vi "ADDER.vi"(2 "INPUT2":bool, 3 "INPUT1":bool) -> (0 "CARRY":bool, 1 "SUM":bool)   [LabVIEW 2017]
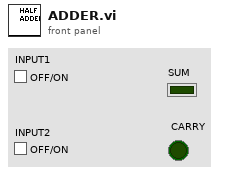
[diagram p1: front panel]
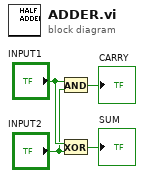
[diagram p0: block diagram]
diagram:
  n1 = And(x="INPUT1", y="INPUT2") -> (x .and. y?=→"CARRY":bool)
  n2 = Exclusive Or(1:"INPUT2", 2:"INPUT1") -> (0:→"SUM":bool)
